vi "Config PLC Tags.vi"(10 "station idx":i32, 11 "configuration file path":path) -> (0 "error out":errorcluster, 2 "PLC Vaule":T1, 3 "configuration file path":path)   [LabVIEW 2018]
uses:
  Crl defs/PLC_bool tags.ctl
  DataSocket/Crl defs/DataSocket_Tags.ctl
  Crl defs/PLC_real tags.ctl
  Crl defs/PLC_string tags.ctl
  Crl defs/one state tags config.ctl
panel:
  in  "string tags":T5
  in  "real tags":T4
  in  "bool tags":T2
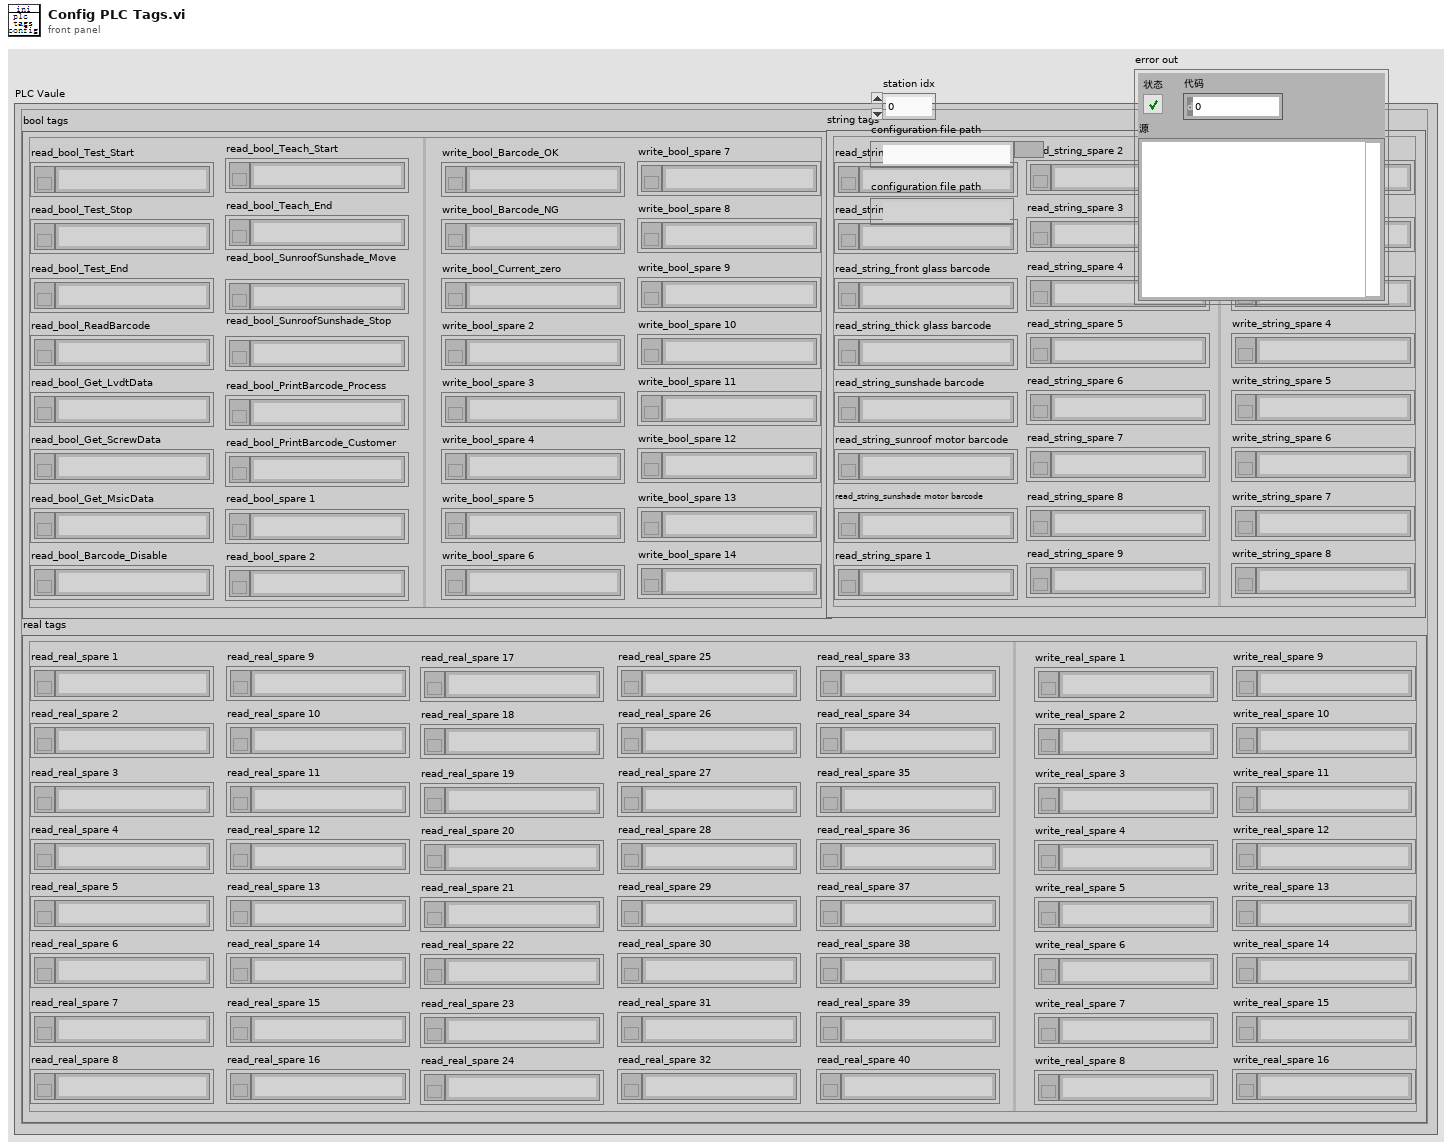
[diagram p1: front panel]
types:
  T1 = typedef "one state tags config.ctl" = cluster{"bool tags":T2, "real tags":T4, "string tags":T5}
  T2 = typedef "PLC_bool tags.ctl" = cluster{"read_bool_Test_Start":T3, "read_bool_Test_Stop":T3, "read_bool_Test_End":T3, "read_bool_ReadBarcode":T3, "read_bool_Get_LvdtData":T3, "read_bool_Get_ScrewData":T3, "read_bool_Get_MsicData":T3, "read_bool_Barcode_Disable":T3, "read_bool_Teach_Start":T3, "read_bool_Teach_End":T3, "read_bool_SunroofSunshade_Move":T3, "read_bool_SunroofSunshade_Stop":T3, "read_bool_PrintBarcode_Process":T3, "read_bool_PrintBarcode_Customer":T3, "read_bool_spare 1":T3, "read_bool_spare 2":T3, "write_bool_Barcode_OK":T3, "write_bool_Barcode_NG":T3, "write_bool_Current_zero":T3, "write_bool_spare 2":T3, "write_bool_spare 3":T3, "write_bool_spare 4":T3, "write_bool_spare 5":T3, "write_bool_spare 6":T3, "write_bool_spare 7":T3, "write_bool_spare 8":T3, "write_bool_spare 9":T3, "write_bool_spare 10":T3, "write_bool_spare 11":T3, "write_bool_spare 12":T3, "write_bool_spare 13":T3, "write_bool_spare 14":T3}
  T3 = typedef "DataSocket_Tags.ctl" = cluster{"Ds ID":refnum<k13>, "Tag":string}
  T4 = typedef "PLC_real tags.ctl" = cluster{"read_real_spare 1":T3, "read_real_spare 2":T3, "read_real_spare 3":T3, "read_real_spare 4":T3, "read_real_spare 5":T3, "read_real_spare 6":T3, "read_real_spare 7":T3, "read_real_spare 8":T3, "read_real_spare 9":T3, "read_real_spare 10":T3, "read_real_spare 11":T3, "read_real_spare 12":T3, "read_real_spare 13":T3, "read_real_spare 14":T3, "read_real_spare 15":T3, "read_real_spare 16":T3, "read_real_spare 17":T3, "read_real_spare 18":T3, "read_real_spare 19":T3, "read_real_spare 20":T3, "read_real_spare 21":T3, "read_real_spare 22":T3, "read_real_spare 23":T3, "read_real_spare 24":T3, "read_real_spare 25":T3, "read_real_spare 26":T3, "read_real_spare 27":T3, "read_real_spare 28":T3, "read_real_spare 29":T3, "read_real_spare 30":T3, "read_real_spare 31":T3, "read_real_spare 32":T3, "read_real_spare 33":T3, "read_real_spare 34":T3, "read_real_spare 35":T3, "read_real_spare 36":T3, "read_real_spare 37":T3, "read_real_spare 38":T3, "read_real_spare 39":T3, "read_real_spare 40":T3, "write_real_spare 1":T3, "write_real_spare 2":T3, "write_real_spare 3":T3, "write_real_spare 4":T3, "write_real_spare 5":T3, "write_real_spare 6":T3, "write_real_spare 7":T3, "write_real_spare 8":T3, "write_real_spare 9":T3, "write_real_spare 10":T3, "write_real_spare 11":T3, "write_real_spare 12":T3, "write_real_spare 13":T3, "write_real_spare 14":T3, "write_real_spare 15":T3, "write_real_spare 16":T3}
  T5 = typedef "PLC_string tags.ctl" = cluster{"read_string_barcode":T3, "read_string_mode type":T3, "read_string_front glass barcode":T3, "read_string_thick glass barcode":T3, "read_string_sunshade barcode":T3, "read_string_sunroof motor barcode":T3, "read_string_sunshade motor barcode\n":T3, "read_string_spare 1":T3, "read_string_spare 2":T3, "read_string_spare 3":T3, "read_string_spare 4":T3, "read_string_spare 5":T3, "read_string_spare 6":T3, "read_string_spare 7":T3, "read_string_spare 8":T3, "read_string_spare 9":T3, "write_string_spare 1":T3, "write_string_spare 2":T3, "write_string_spare 3":T3, "write_string_spare 4":T3, "write_string_spare 5":T3, "write_string_spare 6":T3, "write_string_spare 7":T3, "write_string_spare 8":T3}
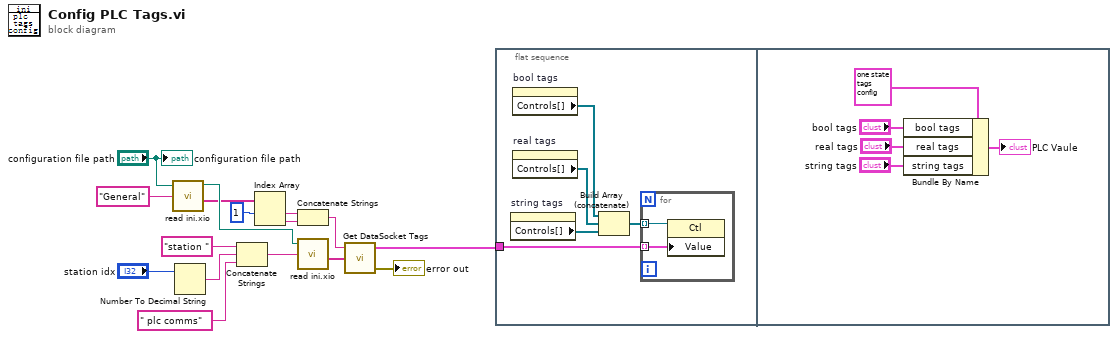
[diagram p0: block diagram]
diagram:
  n1 = call "read ini.xio.vi"("configuration file path"="configuration file path", "Sections"="General") -> ("configuration file path"=w16:path, "Values"=w15:string[])  [unwired: 1 in, 3 out]
  n2 = Number To Decimal String(number="station idx") -> (decimal integer string=w5:string)  [unwired: 1 in]
  n3 = Concatenate Strings("station ", w5, " plc comms" ("string")) -> (w2:string)
  n4 = Index Array(array=w15, index #1=1 ("索引")) -> (element #1=w12:string, element #2=w13:string)  [unwired: 1 in]
  n5 = Concatenate Strings(w12, w13) -> (w11:string)
  n6 = call "read ini.xio.vi"("configuration file path"=w16, "Sections"=w2) -> ("Values"=w7:string[])  [unwired: 1 in, 4 out]
  n7 = call "Get DataSocket Tags.vi"("All Tags"=w7, "URL"=w11) -> ("error out"=→"error out":errorcluster, "DsOut"=w8:T3[])  [unwired: 2 in]
  n8 = flat-sequence {
    tunnel: w8 -> [w17]
    frame #0 {
      n9 = property on="string tags" class="Clust (严格)"() -> ("Controls[]"=w20:refnum<vi>[])  [unwired: 2 in, 2 out]
      n10 = property on="bool tags" class="Clust (严格)"() -> ("Controls[]"=w18:refnum<vi>[])  [unwired: 2 in, 2 out]
      n11 = property on="real tags" class="Clust (严格)"() -> ("Controls[]"=w19:refnum<vi>[])  [unwired: 2 in, 2 out]
      n12 = Build Array (concatenate)(w18, w19, w20) -> (w21:refnum<vi>[])
      n13 = for {
        tunnel: w17 -> [w22] mode=indexing
        tunnel: w21 -> [w23] mode=indexing
        n14 = property class="Ctl"(reference=w23, "Value"=w22) -> ()  [unwired: 1 in, 2 out]
      }
    }
    frame #1 {
      n15 = Bundle By Name(cluster=T1 {"bool tags"={"read_bool_Test_Start"={"Ds ID"=refnum, "Tag"=""}, "read_bool_Test_Stop"={"Ds ID"=refnum, "Tag"=""}, "read_bool_Test_End"={"Ds ID"=refnum, "Tag"=""}, "read_bool_ReadBarcode"={"Ds ID"=refnum, "Tag"=""}, "read_bool_Get_LvdtData"={"Ds ID"=refnum, "Tag"=""}, "read_bool_Get_ScrewData"={"Ds ID"=refnum, "Tag"=""}, "read_bool_Get_MsicData"={"Ds ID"=refnum, "Tag"=""}, "read_bool_Barcode_Disable"={"Ds ID"=refnum, "Tag"=""}, "read_bool_Teach_Start"={"Ds ID"=refnum, "Tag"=""}, "read_bool_Teach_End"={"Ds ID"=refnum, "Tag"=""}, "read_bool_SunroofSunshade_Move"={"Ds ID"=refnum, "Tag"=""}, "read_bool_SunroofSunshade_Stop"={"Ds ID"=refnum, "Tag"=""}, "read_bool_PrintBarcode_Process"={"Ds ID"=refnum, "Tag"=""}, "read_bool_PrintBarcode_Customer"={"Ds ID"=refnum, "Tag"=""}, "read_bool_spare 1"={"Ds ID"=refnum, "Tag"=""}, "read_bool_spare 2"={"Ds ID"=refnum, "Tag"=""}, "write_bool_Barcode_OK"={"Ds ID"=refnum, "Tag"=""}, "write_bool_Barcode_NG"={"Ds ID"=refnum, "Tag"=""}, "write_bool_Current_zero"={"Ds ID"=refnum, "Tag"=""}, "write_bool_spare 2"={"Ds ID"=refnum, "Tag"=""}, "write_bool_spare 3"={"Ds ID"=refnum, "Tag"=""}, "write_bool_spare 4"={"Ds ID"=refnum, "Tag"=""}, "write_bool_spare 5"={"Ds ID"=refnum, "Tag"=""}, "write_bool_spare 6"={"Ds ID"=refnum, "Tag"=""}, "write_bool_spare 7"={"Ds ID"=refnum, "Tag"=""}, "write_bool_spare 8"={"Ds ID"=refnum, "Tag"=""}, "write_bool_spare 9"={"Ds ID"=refnum, "Tag"=""}, "write_bool_spare 10"={"Ds ID"=refnum, "Tag"=""}, "write_bool_spare 11"={"Ds ID"=refnum, "Tag"=""}, "write_bool_spare 12"={"Ds ID"=refnum, "Tag"=""}, "write_bool_spare 13"={"Ds ID"=refnum, "Tag"=""}, "write_bool_spare 14"={"Ds ID"=refnum, "Tag"=""}}, "real tags"={"read_real_spare 1"={"Ds ID"=refnum, "Tag"=""}, "read_real_spare 2"={"Ds ID"=refnum, "Tag"=""}, "read_real_spare 3"={"Ds ID"=refnum, "Tag"=""}, "read_real_spare 4"={"Ds ID"=refnum, "Tag"=""}, "read_real_spare 5"={"Ds ID"=refnum, "Tag"=""}, "read_real_spare 6"={"Ds ID"=refnum, "Tag"=""}, "read_real_spare 7"={"Ds ID"=refnum, "Tag"=""}, "read_real_spare 8"={"Ds ID"=refnum, "Tag"=""}, "read_real_spare 9"={"Ds ID"=refnum, "Tag"=""}, "read_real_spare 10"={"Ds ID"=refnum, "Tag"=""}, "read_real_spare 11"={"Ds ID"=refnum, "Tag"=""}, "read_real_spare 12"={"Ds ID"=refnum, "Tag"=""}, "read_real_spare 13"={"Ds ID"=refnum, "Tag"=""}, "read_real_spare 14"={"Ds ID"=refnum, "Tag"=""}, "read_real_spare 15"={"Ds ID"=refnum, "Tag"=""}, "read_real_spare 16"={"Ds ID"=refnum, "Tag"=""}, "read_real_spare 17"={"Ds ID"=refnum, "Tag"=""}, "read_real_spare 18"={"Ds ID"=refnum, "Tag"=""}, "read_real_spare 19"={"Ds ID"=refnum, "Tag"=""}, "read_real_spare 20"={"Ds ID"=refnum, "Tag"=""}, "read_real_spare 21"={"Ds ID"=refnum, "Tag"=""}, "read_real_spare 22"={"Ds ID"=refnum, "Tag"=""}, "read_real_spare 23"={"Ds ID"=refnum, "Tag"=""}, "read_real_spare 24"={"Ds ID"=refnum, "Tag"=""}, "read_real_spare 25"={"Ds ID"=refnum, "Tag"=""}, "read_real_spare 26"={"Ds ID"=refnum, "Tag"=""}, "read_real_spare 27"={"Ds ID"=refnum, "Tag"=""}, "read_real_spare 28"={"Ds ID"=refnum, "Tag"=""}, "read_real_spare 29"={"Ds ID"=refnum, "Tag"=""}, "read_real_spare 30"={"Ds ID"=refnum, "Tag"=""}, "read_real_spare 31"={"Ds ID"=refnum, "Tag"=""}, "read_real_spare 32"={"Ds ID"=refnum, "Tag"=""}, "read_real_spare 33"={"Ds ID"=refnum, "Tag"=""}, "read_real_spare 34"={"Ds ID"=refnum, "Tag"=""}, "read_real_spare 35"={"Ds ID"=refnum, "Tag"=""}, "read_real_spare 36"={"Ds ID"=refnum, "Tag"=""}, "read_real_spare 37"={"Ds ID"=refnum, "Tag"=""}, "read_real_spare 38"={"Ds ID"=refnum, "Tag"=""}, "read_real_spare 39"={"Ds ID"=refnum, "Tag"=""}, "read_real_spare 40"={"Ds ID"=refnum, "Tag"=""}, "write_real_spare 1"={"Ds ID"=refnum, "Tag"=""}, "write_real_spare 2"={"Ds ID"=refnum, "Tag"=""}, "write_real_spare 3"={"Ds ID"=refnum, "Tag"=""}, "write_real_spare 4"={"Ds ID"=refnum, "Tag"=""}, "write_real_spare 5"={"Ds ID"=refnum, "Tag"=""}, "write_real_spare 6"={"Ds ID"=refnum, "Tag"=""}, "write_real_spare 7"={"Ds ID"=refnum, "Tag"=""}, "write_real_spare 8"={"Ds ID"=refnum, "Tag"=""}, "write_real_spare 9"={"Ds ID"=refnum, "Tag"=""}, "write_real_spare 10"={"Ds ID"=refnum, "Tag"=""}, "write_real_spare 11"={"Ds ID"=refnum, "Tag"=""}, "write_real_spare 12"={"Ds ID"=refnum, "Tag"=""}, "write_real_spare 13"={"Ds ID"=refnum, "Tag"=""}, "write_real_spare 14"={"Ds ID"=refnum, "Tag"=""}, "write_real_spare 15"={"Ds ID"=refnum, "Tag"=""}, "write_real_spare 16"={"Ds ID"=refnum, "Tag"=""}}, "string tags"={"read_string_barcode"={"Ds ID"=refnum, "Tag"=""}, "read_string_mode type"={"Ds ID"=refnum, "Tag"=""}, "read_string_front glass barcode"={"Ds ID"=refnum, "Tag"=""}, "read_string_thick glass barcode"={"Ds ID"=refnum, "Tag"=""}, "read_string_sunshade barcode"={"Ds ID"=refnum, "Tag"=""}, "read_string_sunroof motor barcode"={"Ds ID"=refnum, "Tag"=""}, "read_string_sunshade motor barcode\n"={"Ds ID"=refnum, "Tag"=""}, "read_string_spare 1"={"Ds ID"=refnum, "Tag"=""}, "read_string_spare 2"={"Ds ID"=refnum, "Tag"=""}, "read_string_spare 3"={"Ds ID"=refnum, "Tag"=""}, "read_string_spare 4"={"Ds ID"=refnum, "Tag"=""}, "read_string_spare 5"={"Ds ID"=refnum, "Tag"=""}, "read_string_spare 6"={"Ds ID"=refnum, "Tag"=""}, "read_string_spare 7"={"Ds ID"=refnum, "Tag"=""}, "read_string_spare 8"={"Ds ID"=refnum, "Tag"=""}, "read_string_spare 9"={"Ds ID"=refnum, "Tag"=""}, "write_string_spare 1"={"Ds ID"=refnum, "Tag"=""}, "write_string_spare 2"={"Ds ID"=refnum, "Tag"=""}, "write_string_spare 3"={"Ds ID"=refnum, "Tag"=""}, "write_string_spare 4"={"Ds ID"=refnum, "Tag"=""}, "write_string_spare 5"={"Ds ID"=refnum, "Tag"=""}, "write_string_spare 6"={"Ds ID"=refnum, "Tag"=""}, "write_string_spare 7"={"Ds ID"=refnum, "Tag"=""}, "write_string_spare 8"={"Ds ID"=refnum, "Tag"=""}}} ("all tags of plc"), "bool tags"="bool tags", "real tags"="real tags", "string tags"="string tags") -> (→"PLC Vaule":T1)
    }
  }
  "configuration file path" <- "configuration file path"
